vi "get_status_power.vi"(8 "error in (no error)":errorcluster, 11 "LightSourceAN191011Chameleon in":refnum<class "LightSourceAN191011Chameleon.lvclass">) -> (0 "error out":errorcluster, 2 "output power":dbl[unit], 3 "LightSourceAN191011Chameleon out":refnum<class "LightSourceAN191011Chameleon.lvclass">)   [LabVIEW 2011, in "LightSourceAN191011Chameleon.lvclass"]
uses:
  LightSourceAN191011Chameleon.lvclass
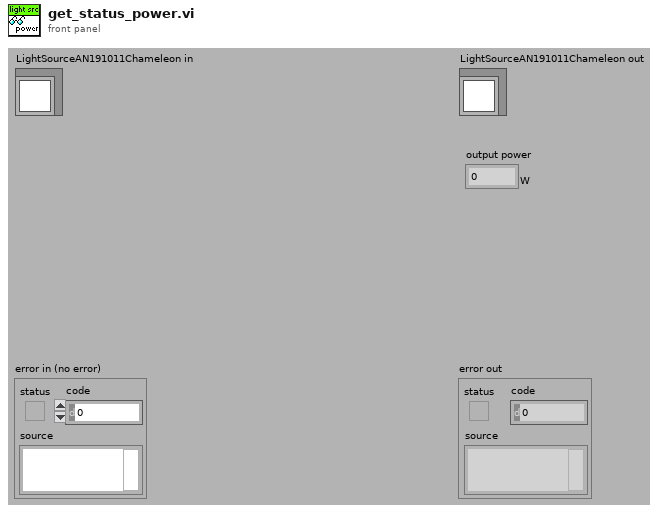
[diagram p1: front panel]
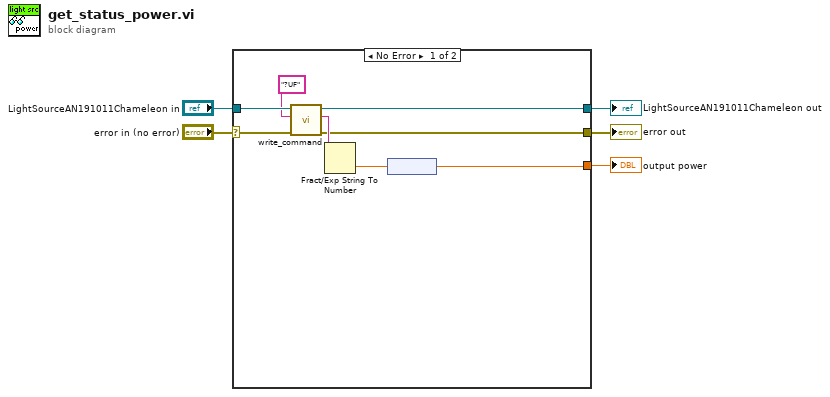
[diagram p0: block diagram]
diagram:
  n1 = case shown="No Error" "error in (no error)" {
    selector: "error in (no error)" -> [w12 w15]
    tunnel: [w6 w15] -> w4
    tunnel: [w8 w14] -> w2
    tunnel: "LightSourceAN191011Chameleon in" -> [w13 w14]
    tunnel: [w7 _] -> w1
    frame No Error {
      n2 = call-dynamic "write_command.vi"("error in (no error)"=w12, "string to write"="?UF", "LightSourceAN191011Chameleon in"=w13) -> ("error out"=w6:errorcluster, "read string"=w10:string, "LightSourceAN191011Chameleon out"=w8:refnum<class "LightSourceAN191011Chameleon.lvclass">)  [unwired: 6 in]
      n3 = Fract/Exp String To Number(string=w10) -> (number=w9:dbl)  [unwired: 3 in, 1 out]
      n4 = node(w9) -> (w7:dbl[unit])
    }
    frame Error {
    }
  }
  "error out" <- w4
  "LightSourceAN191011Chameleon out" <- w2
  "output power" <- w1
